vi "NewWall.vi"(8 "error in (no error)":errorcluster) -> (0 "error out":errorcluster, 3 "Wall":refnum<class "Wall.lvclass">)   [LabVIEW 2020, in "Wall.lvclass"]
uses:
  Wall.lvclass
  Support/Class/ConsoleOutput.lvclass
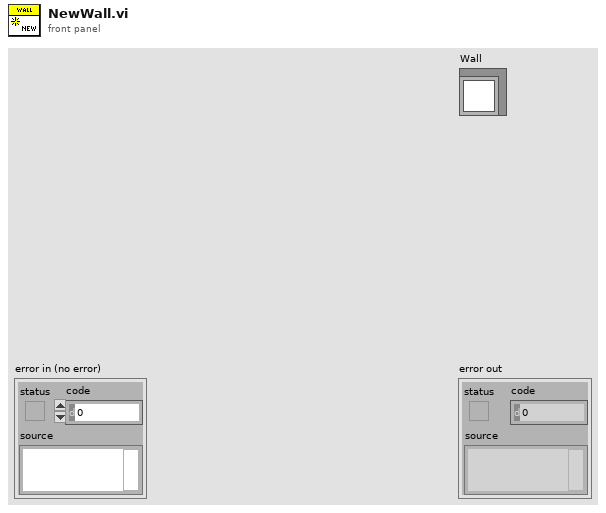
[diagram p1: front panel]
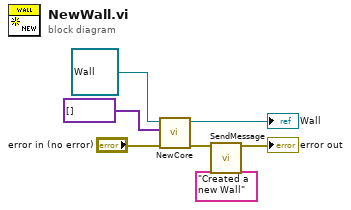
[diagram p0: block diagram]
diagram:
  n1 = call-dynamic "NewCore.vi"("error in (no error)"="error in (no error)", "ParamsArray"=variant[] [], "Room"=refnum<class "Wall.lvclass"> refnum ("ByRef")) -> ("error out"=w2:errorcluster, "Room"=→"Wall":refnum<class "Wall.lvclass">)  [unwired: 7 in]
  n2 = call "SendMessage.vi"("Message"="Created a new Wall", "error in (no error)"=w2) -> ("error out"=→"error out":errorcluster)  [unwired: 13 in]
